vi "Format Variant Attributes into String.vi"(8 "error in (no error)":errorcluster, 11 "Variant":variant) -> (0 "error out":errorcluster, 3 "Data":string)   [LabVIEW 2017]
doc: "Formats every attribute of the Variant into a readable string of the form VariantAttributes(name0 -> value0;name1 -> value1;...)."
uses:
  _openG/_reuse_openG.lvlib
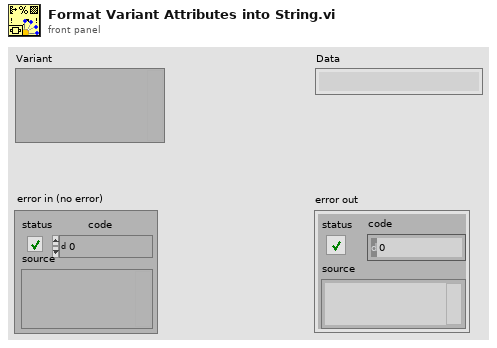
[diagram p1: front panel]
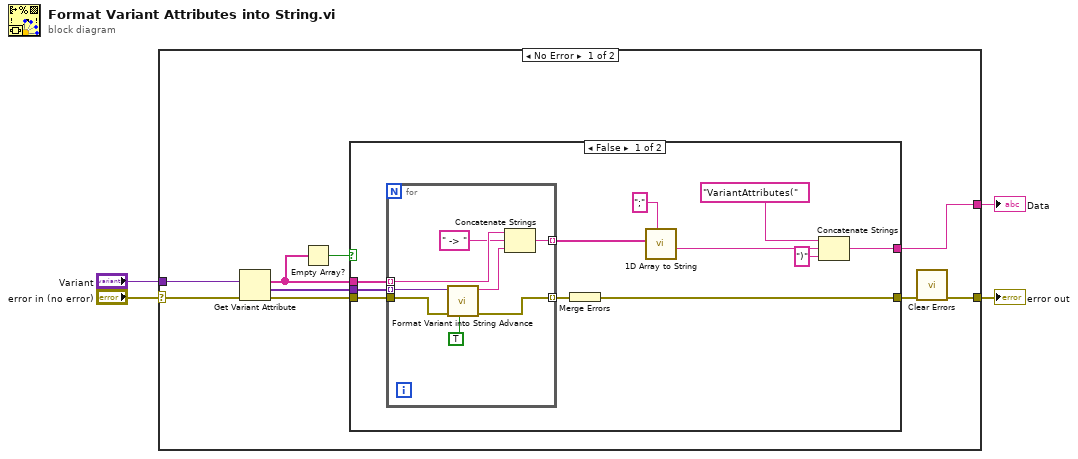
[diagram p0: block diagram]
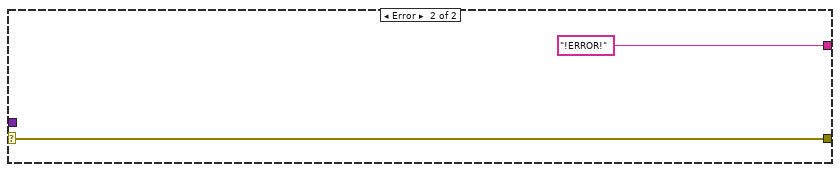
[diagram p3: hidden frame]
diagram:
  n1 = case shown="No Error" "error in (no error)" {
    selector: "error in (no error)" -> [w13 w35]
    tunnel: [w5 "!ERROR!" ("Output String")] -> w4
    tunnel: [w12 w35] -> w2
    tunnel: "Variant" -> [w11 _]
    frame No Error {
      n2 = Get Variant Attribute(Variant=w11, error in=w13) -> (names=w8:string[], values=w9:variant[], error out=w7:errorcluster)  [unwired: 2 in, 1 out]
      n3 = Empty Array?(array=w8) -> (empty?=w6:bool)
      n4 = case shown="False" w6 {
        tunnel: w9 -> [w24 _]
        tunnel: w8 -> [w23 _]
        tunnel: w7 -> [w22 w33]
        tunnel: [w20 w33] -> w10
        tunnel: [w16 _] -> w5
        frame False {
          n5 = for {
            tunnel: w23 -> [w29] mode=indexing
            tunnel: w24 -> [w32] mode=indexing
            tunnel: w22 -> [w31]
            tunnel: [w30] -> w21 mode=indexing
            tunnel: [w26] -> w19 mode=indexing
            n6 = call "Format Variant into String Advance.vi"("include Variant Attributes(F)"=TRUE ("include Variant Attributes"), "error in (no error)"=w31, "Variant"=w32) -> ("error out"=w30:errorcluster, "Data"=w28:string)  [unwired: 6 in, 1 out]
            n7 = Concatenate Strings(w29, " -> " ("string"), w28) -> (w26:string)
          }
          n8 = Merge Errors(w21) -> (w20:errorcluster)
          n9 = call "1D Array to String.vi"("delimiter (Tab)"=";", "Array of Strings"=w19) -> ("delimited string"=w17:string)  [unwired: 9 in]
          n10 = Concatenate Strings("VariantAttributes(" ("string"), w17, ")" ("string")) -> (w16:string)
        }
        frame True {
        }
      }
      n11 = call <vilib>:"Clear Errors.vi"("error in (no error)"=w10) -> ("error out"=w12:errorcluster)  [unwired: 5 in, 1 out]
    }
    frame Error {
    }
  }
  "Data" <- w4
  "error out" <- w2
